vi "interlock_with_heat_ex_top.vi"(6 "limit":dbl=1400.0, 7 "enable_interlock":bool caption="Interlock", 8 "turn_max":dbl=0.5, 9 "ref_sp_bv_turn":refnum<vi>, 10 "ref_sp_rv_turn":refnum<vi>) -> (0 "status":u32(colorbox)=9567230)   [LabVIEW 2019]
doc: "This example demonstrates how to simulate a general PID controller."
uses:
  LakeShore218/LakeShore218_Global.vi
panel:
  out "value":dbl
  # "Ohm"
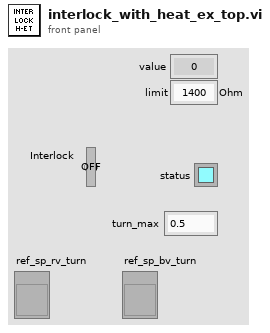
[diagram p1: front panel]
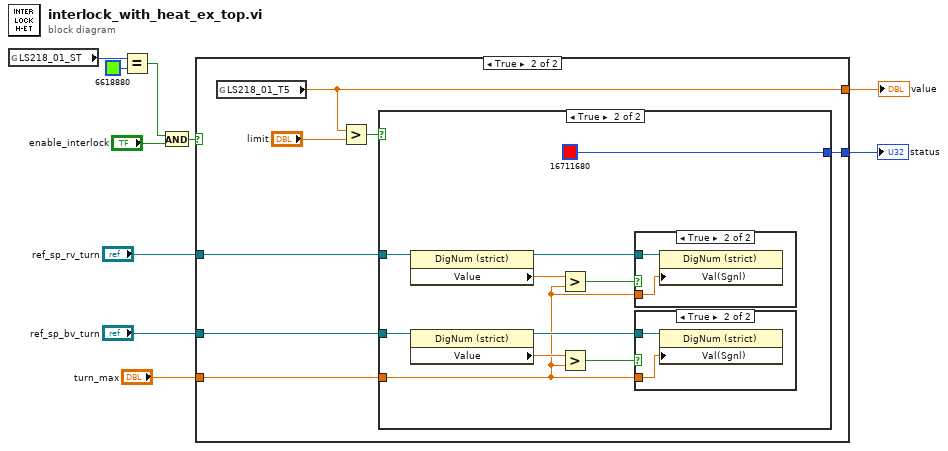
[diagram p0: block diagram]
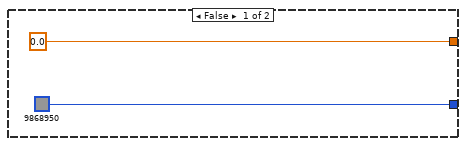
[diagram p2: hidden frame]
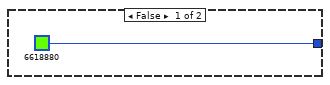
[diagram p3: hidden frame]
diagram:
  n1 = global read "LakeShore218_Global.vi" "LS218_01_ST"() -> (w3:u32)
  n2 = Equal?(x=w3, y=u32 6618880 ("alarm_status")) -> (x = y?=w1:bool)
  n3 = And(x=w1, y="enable_interlock") -> (x .and. y?=w7:bool)
  n4 = case shown="True" w7 {
    tunnel: [u32 9868950 ("alarm_status") w19] -> w10
    tunnel: [0.0 ("Value") w13] -> w9
    tunnel: "ref_sp_rv_turn" -> [_ w17]
    tunnel: "turn_max" -> [_ w15]
    tunnel: "ref_sp_bv_turn" -> [_ w14]
    frame False {
    }
    frame True {
      n5 = global read "LakeShore218_Global.vi" "LS218_01_T5"() -> (w13:dbl)
      n6 = Greater?(x=w13, y="limit") -> (0:w16:bool)
      n7 = case shown="True" w16 {
        tunnel: [u32 6618880 ("alarm_status") u32 16711680 ("alarm_status")] -> w19
        tunnel: w17 -> [_ w29]
        tunnel: w15 -> [_ w21]
        tunnel: w14 -> [_ w25]
        frame False {
        }
        frame True {
          n8 = property class="DigNum (strict)"(reference=w29) -> (reference out=w26:refnum<vi>, "Value"=w28:dbl)  [unwired: 1 in, 1 out]
          n9 = property class="DigNum (strict)"(reference=w25) -> (reference out=w22:refnum<vi>, "Value"=w24:dbl)  [unwired: 1 in, 1 out]
          n10 = Greater?(x=w28, y=w21) -> (0:w27:bool)
          n11 = Greater?(x=w24, y=w21) -> (0:w23:bool)
          n12 = case shown="True" w27 {
            tunnel: w26 -> [_ w34]
            tunnel: w21 -> [_ w33]
            frame False {
            }
            frame True {
              n13 = property class="DigNum (strict)"(reference=w34, "Val(Sgnl)"=w33) -> ()  [unwired: 1 in, 2 out]
            }
          }
          n14 = case shown="True" w23 {
            tunnel: w22 -> [_ w32]
            tunnel: w21 -> [_ w31]
            frame False {
            }
            frame True {
              n15 = property class="DigNum (strict)"(reference=w32, "Val(Sgnl)"=w31) -> ()  [unwired: 1 in, 2 out]
            }
          }
        }
      }
    }
  }
  "status" <- w10
  "value" <- w9
